vi "Queue Comms Enqueue.vi"(8 "error in (no error)":errorcluster, 11 "element":T1={"Data"=variant, "Action"=enum."Init"}) -> (0 "error out":errorcluster)   [LabVIEW 2018, in "File IO.lvlib"]
doc: "This subVI enqueues an element in to the communications queue to be handled"
uses:
  File IO.lvlib
  Private Controls/Module Data.ctl
  Private Controls/Module Action.ctl
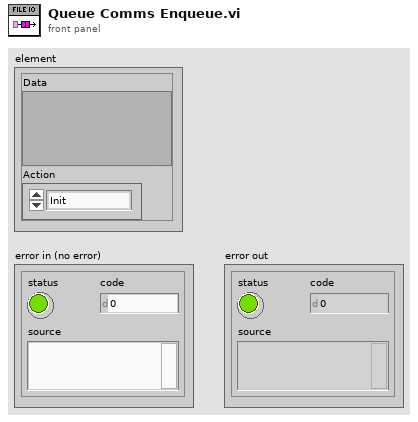
[diagram p1: front panel]
types:
  T1 = typedef "File IO.lvlib/Module Data.ctl" = cluster{"Data":variant, "Action":T2}
  T2 = typedef "File IO.lvlib/Module Action.ctl" = enum8{"Timeout", "OpenReport", "Continue Test", "Init", "Error", "Exit", "Save Accel Data", "Set Recording State", "Log APU RunTime", "Start New Test", "Create New Reports", "Write to System Log", "Save Variables", "Load APU Setup File", "Increment Run Count", "Write To Report"}
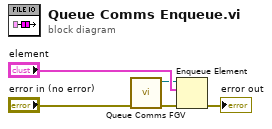
[diagram p0: block diagram]
diagram:
  n1 = call "Queue Comms FGV.vi"("error in (no error)"="error in (no error)") -> ("error out"=w4:errorcluster, "Queue out"=w2:refnum<queue>)  [unwired: 9 in]
  n2 = Enqueue Element(queue=w2, element="element", error in (no error)=w4) -> (error out=→"error out":errorcluster)  [unwired: 1 in, 2 out]
